vi "test_00_temp.vi"() -> ()   [LabVIEW 2015, in "lv-unit-conversion.lvlib"]
uses:
  lv-unit-conversion.lvlib
panel:
  out "value out":dbl
  in  "value in":dbl
  in  "from_unit":string="m"
  in  "to_unit":string="in"
  out "data_set":variant
  out "error out":errorcluster
  in  "error in (no error)":errorcluster
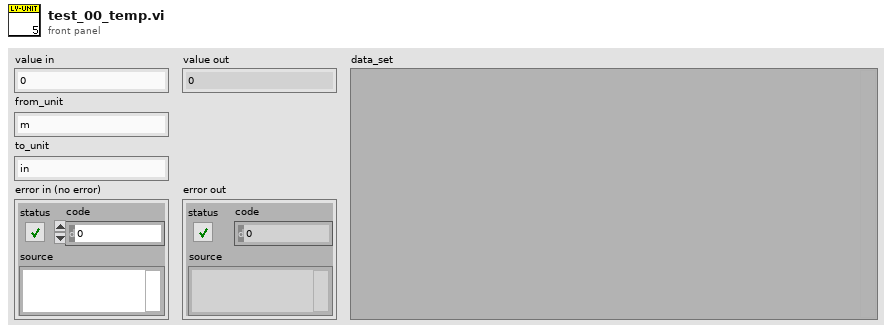
[diagram p1: front panel]
types:
  T1 = typedef "lv-unit-conversion.lvlib/unit_set.ctl" = cluster{"symbol":string, "name":string, "dimension":string, "is_si_unit":bool, "category":string, "base_unit":string, "conversion_reference":string, "is_exact":bool, "a":dbl, "b":dbl, "c":dbl, "d":dbl, "underlying_def":string, "description":string}
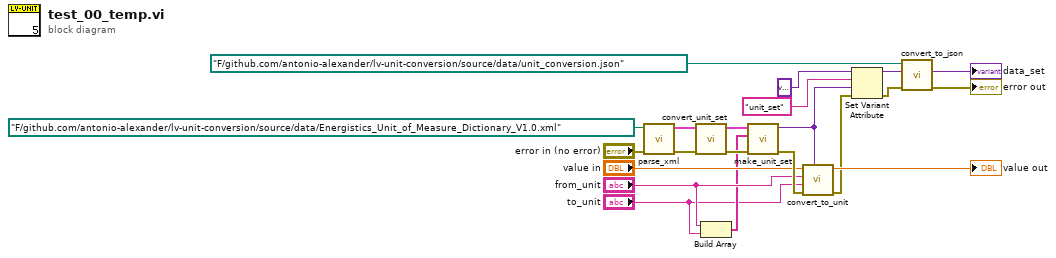
[diagram p0: block diagram]
diagram:
  n1 = call "parse_xml.vi"("error in (no error)"="error in (no error)", "XML File Path"=path "F:/github.com/antonio-alexander/lv-unit-conversion/source/data/Energistics_Unit_of_Measure_Dictionary_V1.0.xml") -> ("error out"=w18:errorcluster, "raw_data []"=w19:cluster{"Name":string, cluster{cluster[]}[]}[])  [unwired: 8 in]
  n2 = call "convert_unit_set.vi"("error in (no error)"=w18, "raw_data []"=w19) -> ("error out"=w14:errorcluster, "units []"=w15:T1[])  [unwired: 8 in]
  n3 = Build Array("from_unit", "to_unit") -> (w10:string[])
  n4 = call "make_unit_set.vi"("error in (no error)"=w14, "symbols []"=w10, "units []"=w15) -> ("error out"=w20:errorcluster, "unit_set out"=w6:variant)  [unwired: 7 in]
  n5 = call "convert_to_unit.vi"("unit_set"=w6, "error in (no error)"=w20, "unit_to"="to_unit", "unit_from"="from_unit", "value in"="value in") -> ("error out"=w5:errorcluster, "value out"=→"value out":dbl)  [unwired: 5 in]
  n6 = Set Variant Attribute(Variant=variant, name="unit_set", value=w6, error in=w5) -> (Variant out=w4:variant, error out=w3:errorcluster)  [unwired: 1 out]
  "data_set" <- w4
  n7 = call "convert_to_json.vi"("error in (no error)"=w3, "data_set"=w4, "json_path"=path "F:/github.com/antonio-alexander/lv-unit-conversion/source/data/unit_conversion.json") -> ("error out"=→"error out":errorcluster)  [unwired: 8 in]
